vi "ClassPanel.vi"(8 "error in (no error)":errorcluster caption="entrée d'erreur (pas d'erreur)", 11 "BNC845.lvclass":refnum<class "BNC845.lvclass">) -> (0 "error out":errorcluster caption="sortie d'erreur", 3 "BNC845.lvclass Out":refnum<class "BNC845.lvclass">)   [LabVIEW 2019, in "BNC845.lvclass"]
uses:
  BNC845.lvclass
  C:/Programmes Labview/LabscanV1A/DevicesClass/BaseDevice/BaseDevice.lvclass
  BaseDevice/ClassQueueMess.ctl
  BNC845_Func.ctl
  BNC845.lvclass/BNC845.ctl
  BaseDevice/Accessor/GetClassEvent.vi
  <instrlib>/Berkeley Nucleonics 845/Berkeley Nucleonics 845.lvlib
panel:
  in  "Scan Mode":u16(ring) items=["Frequency", "Power"]
  in  "Output En":bool
  in  "Con/Disc.":bool
  in  "FUnits":u16(ring)=1 caption="Units" items=["Hz", "MHz", "GHz"]
  in  "MainProgQ":refnum<queue>
  in  "MainProgQEvent":refnum<user-event>
  in  "Acq":bool
  in  "Stop":bool
  in  "Power":dbl caption="Power(dBm)" format="%#.3f"
  in  "MiseAJour":bool
  in  "Freq(Hz)":dbl=60.0 min=0.01 max=20500000000.0 step=0.01 format="%^#.5e"
  out "Init Program":bool
  # "BNC845"
  # "this MUST labeled with class name"
  # "this MUST be present and labeled \"Stop\" and \"Acq\""
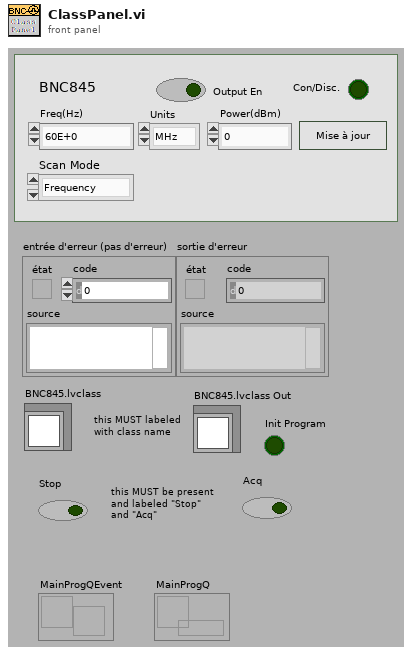
[diagram p1: front panel]
types:
  T1 = typedef "BNC845.lvclass/BNC845_Func.ctl" = enum16{"SetPower (dBm)", "SetFrequency (Hz)"}
  T2 = typedef "ClassQueueMess.ctl" = u16
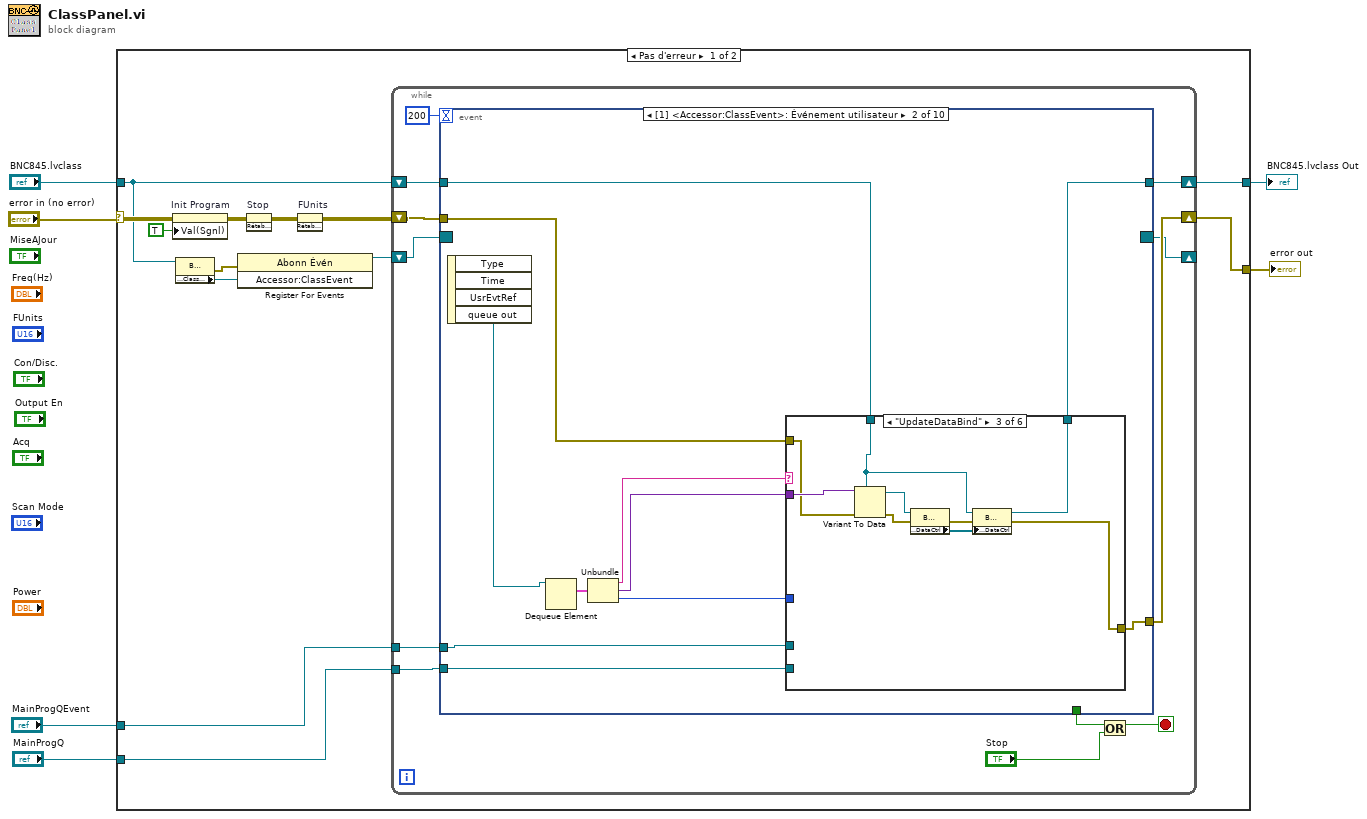
[diagram p0: block diagram]
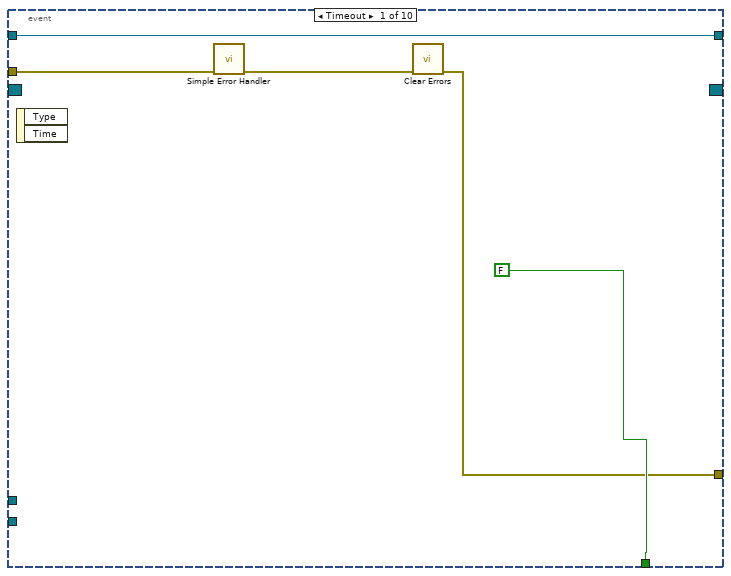
[diagram p2: hidden frame]
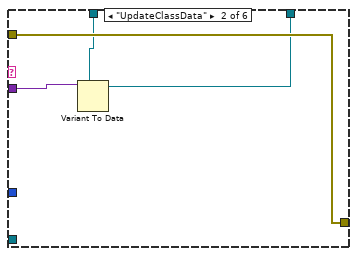
[diagram p4: hidden frame]
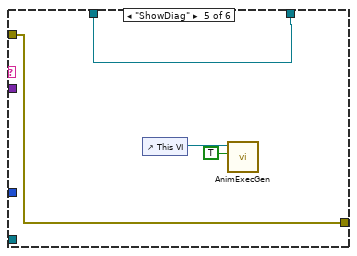
[diagram p6: hidden frame]
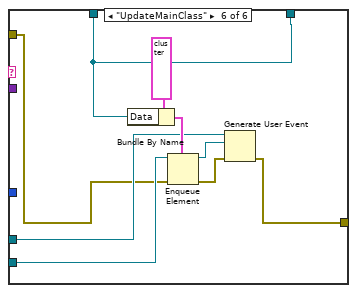
[diagram p7: hidden frame]
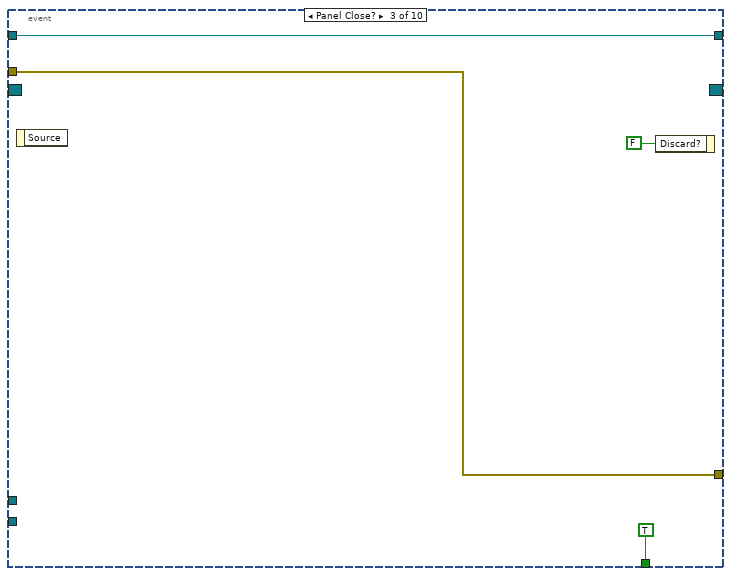
[diagram p8: hidden frame]
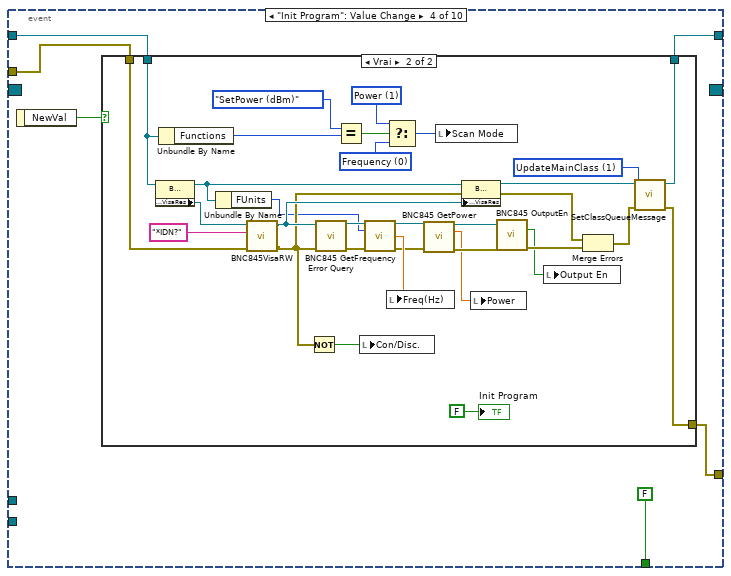
[diagram p9: hidden frame]
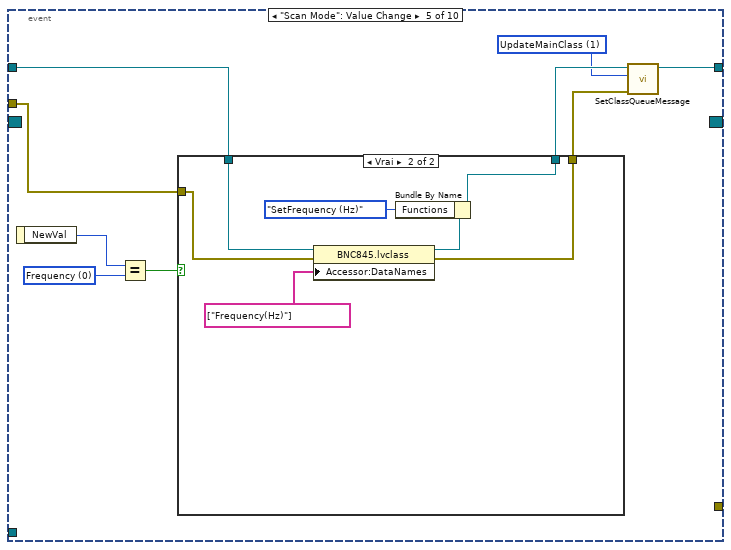
[diagram p11: hidden frame]
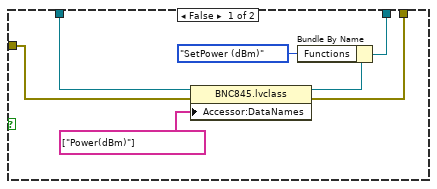
[diagram p12: hidden frame]
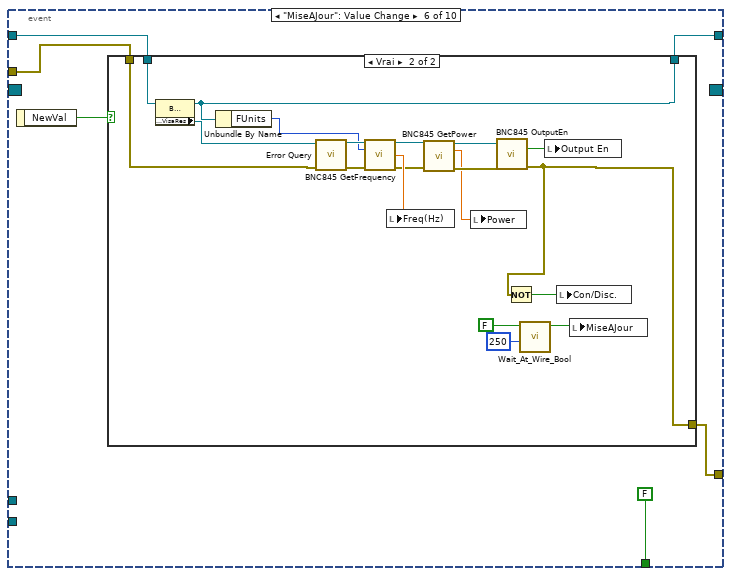
[diagram p13: hidden frame]
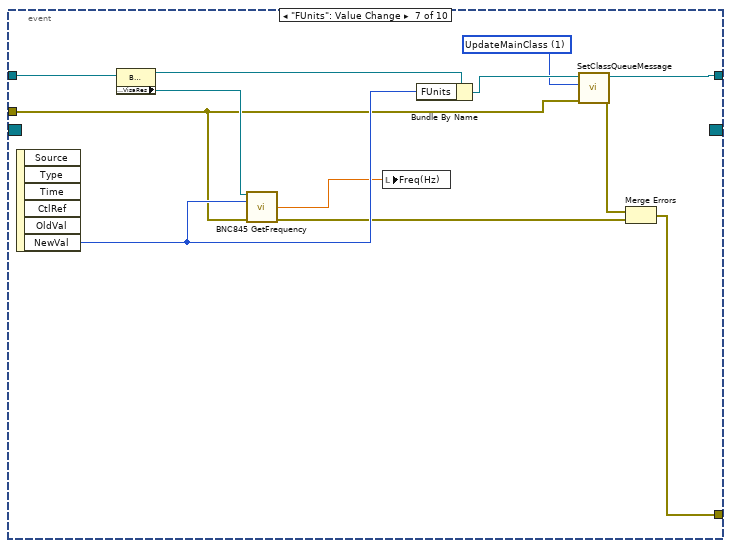
[diagram p15: hidden frame]
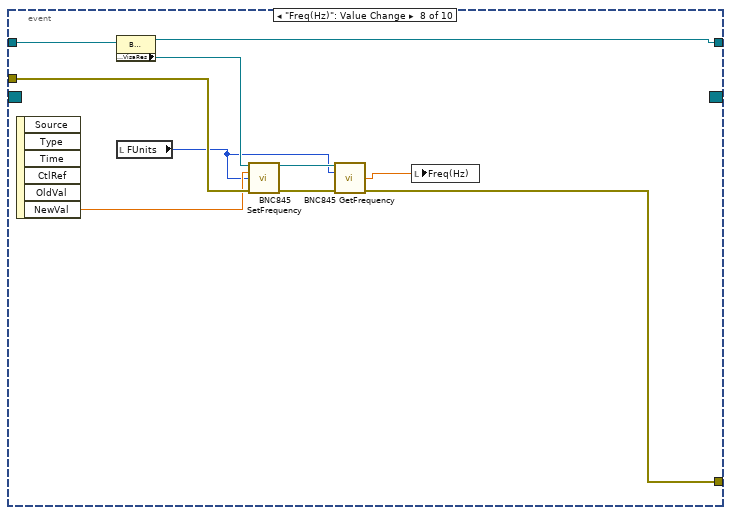
[diagram p16: hidden frame]
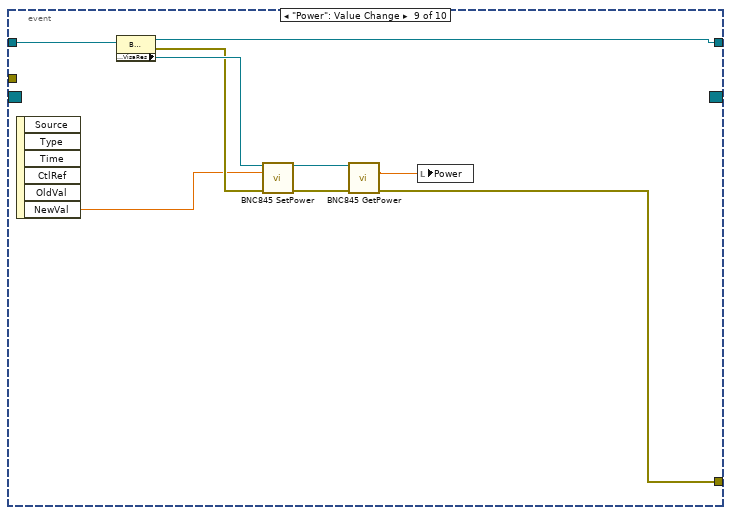
[diagram p17: hidden frame]
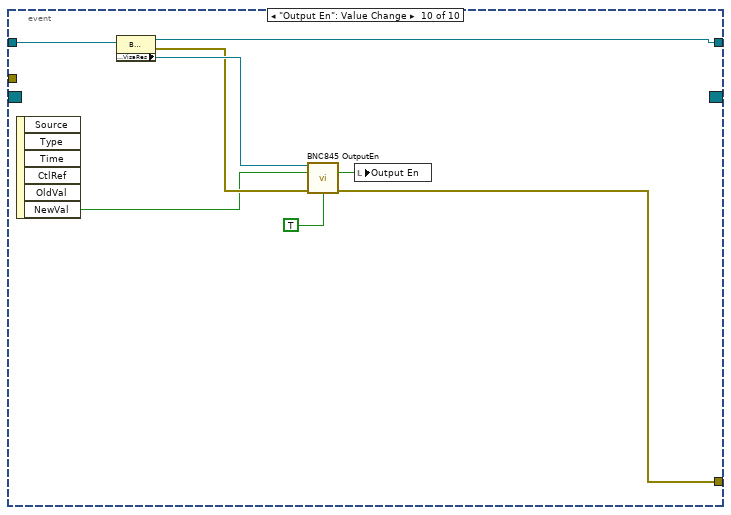
[diagram p18: hidden frame]
diagram:
  n1 = case shown="Pas d'erreur" "error in (no error)" {
    selector: "error in (no error)" -> [w16 w212]
    tunnel: [w19 w212] -> w5
    tunnel: "BNC845.lvclass" -> [w12 w211]
    tunnel: [w17 w211] -> w3
    tunnel: "MainProgQEvent" -> [w10 _]
    tunnel: "MainProgQ" -> [w9 _]
    frame No Error {
      n2 = property on="Init Program" class="Bool (strict)"(error in=w16, "Val(Sgnl)"=TRUE ("Valeur (Signalisation)")) -> (error out=w15:errorcluster)  [unwired: 1 in, 1 out]
      n3 = property class="BNC845.lvclass"(reference=w12) -> (error out=w14:errorcluster, "Accessor:ClassEvent"=w13:refnum<user-event>)  [unwired: 1 in, 1 out]
      n4 = register-events(error in=w14, w13) -> (reference out=w11:refnum<event-registration>)  [unwired: 1 in, 1 out]
      n5 = invoke on="Stop" class="Bool (strict)" method="RétablirValParDéfaut"(error in=w15) -> (error out=w8:errorcluster)  [unwired: 2 in, 2 out]
      n6 = invoke on="FUnits" class="MDér (strict)" method="RétablirValParDéfaut"(error in=w8) -> (error out=w7:errorcluster)  [unwired: 2 in, 2 out]
      n7 = while {
        shift-right: [w29] -> w19
        shift-left: w7 -> [w30]
        shift-right: [w26] -> w17
        shift-left: w12 -> [w28]
        shift-right: [w22] -> _
        shift-left: w11 -> [w23]
        tunnel: w10 -> [w21]
        tunnel: w9 -> [w20]
        stop <- w25 stop-if-true
        n8 = event shown="[1] <Accessor:ClassEvent>: Événement utilisateur" {
          selector: w23 -> [_ _ _ _ _ _ _ _ _ _]
          dyn-events: [_ _ _ _ _ _ _ _ _ _] -> w22
          timeout: 200 -> [_ _ _ _ _ _ _ _ _ _]
          tunnel: w30 -> [w34 w46 w79 w86 w124 w149 w177 w191 _ _]
          tunnel: [w32 w40 w79 w85 _ w148 w175 w185 w199 w208] -> w29
          tunnel: w28 -> [w35 w47 w78 w83 w126 w146 w183 w193 w202 w210]
          tunnel: [FALSE _ TRUE FALSE _ FALSE _ _ _ _] -> w27
          tunnel: [w35 w39 w78 w82 w127 w145 w173 w192 w201 w209] -> w26
          tunnel: w21 -> [_ w38 _ _ _ _ _ _ _ _]
          tunnel: w20 -> [_ w37 _ _ _ _ _ _ _ _]
          event Timeout {
            n9 = event-data() -> ()  [unwired: 1 in, 2 out]
            n10 = call <vilib>:"Simple Error Handler.vi"("error in (no error)"=w34) -> ("error out"=w33:errorcluster)  [unwired: 4 in, 4 out]
            n11 = call <vilib>:"Clear Errors.vi"("error in (no error)"=w33) -> ("error out"=w32:errorcluster)  [unwired: 5 in, 1 out]
          }
          event User Event {
            n12 = event-data() -> ("queue out"=w44:refnum<queue>)  [unwired: 1 in, 3 out]
            n13 = Dequeue Element(queue=w44) -> (element=w45:cluster{"Message":string, "Data":variant, i32})  [unwired: 2 in, 3 out]
            n14 = Unbundle(w45) -> ("Message"=w43:string, "Data"=w42:variant, w41:i32)
            n15 = case shown="\"UpdateDataBind\"" w43 {
              tunnel: w46 -> [w49 w53 w54 w63 w67 w70]
              tunnel: w42 -> [_ w52 w62 _ _ _]
              tunnel: w47 -> [w48 w51 w58 w64 w68 w73]
              tunnel: [w48 w50 w57 w64 w68 w73] -> w39
              tunnel: [w49 w53 w55 w63 w67 w69] -> w40
              tunnel: w41 -> [_ _ _ _ _ _]
              tunnel: w38 -> [_ _ _ _ _ w72]
              tunnel: w37 -> [_ _ _ _ _ w71]
              frame Default {
              }
              frame "UpdateClassData" {
                n16 = Variant To Data(type=w51, Variant=w52) -> (data=w50:refnum<class "BNC845.lvclass">)  [unwired: 1 in, 1 out]
              }
              frame "UpdateDataBind" {
                n17 = Variant To Data(error in=w54, type=w58, Variant=w62) -> (data=w59:refnum<class "BNC845.lvclass">, error out=w56:errorcluster)
                n18 = property class="BNC845.lvclass"(reference=w59, error in=w56) -> (error out=w61:errorcluster, "Accessor:DataCtrl"=w60:refnum<vi>[])  [unwired: 1 out]
                n19 = property class="BNC845.lvclass"(reference=w58, error in=w61, "Accessor:DataCtrl"=w60) -> (reference out=w57:refnum<class "BNC845.lvclass">, error out=w55:errorcluster)
              }
              frame "MeasDone" {
              }
              frame "ShowDiag" {
                n20 = control-ref of="This VI"() -> (w66:refnum<vi>)
                n21 = call <userlib>:"AnimExecGen.vi"("Animer l'exécution ?"=TRUE, "ViRef"=w66) -> ()  [unwired: 9 in, 1 out]
              }
              frame "UpdateMainClass" {
                n22 = Bundle By Name(cluster=cluster{"Message":string, "Data":variant, i32} {"Message"="", "Data"=variant, 0} ("élément"), "Data"=w73) -> (w74:cluster{"Message":string, "Data":variant, i32})
                n23 = Enqueue Element(queue=w71, element=w74, error in (no error)=w70) -> (queue out=w77:refnum<queue>, error out=w76:errorcluster)  [unwired: 1 in, 1 out]
                n24 = Generate User Event(user event=w72, event data cluster=w77, error in=w76) -> (error out=w69:errorcluster)  [unwired: 1 in, 1 out]
              }
            }
          }
          event Panel Close? {
            n25 = event-data() -> ()  [unwired: 1 in, 1 out]
            n26 = event-data("Discard?"=FALSE ("Rejeter ?")) -> ()  [unwired: 1 in, 1 out]
          }
          event "Init Program": Value Change {
            n27 = event-data() -> ("NewVal"=w87:bool)  [unwired: 1 in]
            n28 = case shown="Vrai" w87 {
              tunnel: w86 -> [w89 w119]
              tunnel: [w89 w103] -> w85
              tunnel: w83 -> [w88 w96]
              tunnel: [w88 w108] -> w82
              frame False {
              }
              frame True {
                w90 = u16 0 items=["Frequency", "Power"] ("Scan Mode")
                w91 = u16 1 items=["Frequency", "Power"] ("Scan Mode")
                w107 = T2 1 items=["UpdateClassData", "UpdateMainClass", "UpdateDataBind", "ReInitDevice", "Custom", "ClosePan"] ("Menu déroulant")
                n29 = property class="BNC845.lvclass"(reference=w96) -> (reference out=w111:refnum<class "BNC845.lvclass">, "Accessor:VisaRes"=w120:refnum<visa-resource-name>)  [unwired: 1 in, 1 out]
                n30 = Unbundle By Name(w96) -> ("Functions"=w94:T1)
                n31 = Unbundle By Name(w111) -> ("FUnits"=w110:u16)
                n32 = call <instrlib>:"BNC845VisaRW.vi"("error in (no error)"=w119, "ChaineCom"="*IDN?", "VISA Rsrc"=w120) -> ("error out"=w114:errorcluster, "VISA Rsrc Out"=w115:refnum<visa-resource-name>)  [unwired: 4 in, 2 out]
                n33 = Not(x=w114) -> (.not. x?=w113:bool)
                n34 = call <instrlib>:"Error Query.vi"("VISA resource name"=w115, "error in (no error)"=w114) -> ("VISA resource name out"=w116:refnum<visa-resource-name>, "error out"=w117:errorcluster)  [unwired: 10 in, 2 out]
                n35 = Equal?(x=BNC845_Func."SetPower (dBm)" ("Functions"), y=w94) -> (x = y?=w93:bool)
                n36 = local write "Con/Disc."(w113) -> ()
                n37 = call <instrlib>:"BNC845 GetFrequency.vi"("VISA Rsrc"=w116, "FUnits"=w110, "error in (no error)"=w117) -> ("VISA Rsrc Out"=w101:refnum<visa-resource-name>, "Frequency (Units)"=w112:dbl, "error out"=w102:errorcluster)  [unwired: 9 in, 1 out]
                n38 = Select(t=w91, s=w93, f=w90) -> (s? t:f=w92:u16)
                n39 = local write "Freq(Hz)"(w112) -> ()
                n40 = call <instrlib>:"BNC845 GetPower.vi"("VISA Rsrc"=w101, "error in (no error)"=w102) -> ("VISA Rsrc Out"=w98:refnum<visa-resource-name>, "Power (dBm)"=w99:dbl, "error out"=w100:errorcluster)  [unwired: 11 in]
                n41 = local write "Scan Mode"(w92) -> ()
                n42 = property class="BNC845.lvclass"(reference=w111, error in=w114, "Accessor:VisaRes"=w115) -> (reference out=w106:refnum<class "BNC845.lvclass">, error out=w105:errorcluster)
                n43 = local write "Power"(w99) -> ()
                n44 = call <instrlib>:"BNC845 OutputEn.vi"("VISA Rsrc"=w98, "error in (no error)"=w100) -> ("Enabled"=w97:bool, "error out"=w109:errorcluster)  [unwired: 11 in, 1 out]
                n45 = local write "Output En"(w97) -> ()
                n46 = Merge Errors(w105, w109) -> (w104:errorcluster)
                n47 = call-dynamic "SetClassQueueMessage.vi"("ErrorIn(No Error)"=w104, "Menu déroulant"=w107, "DefaultDev.lvclass"=w106) -> ("sortie d'erreur"=w103:errorcluster, "DefaultDev.lvclass Out"=w108:refnum<class "BNC845.lvclass">)  [unwired: 7 in]
                "Init Program" <- FALSE
              }
            }
          }
          event "Scan Mode": Value Change {
            w122 = T2 1 items=["UpdateClassData", "UpdateMainClass", "UpdateDataBind", "ReInitDevice", "Custom", "ClosePan"] ("Menu déroulant")
            w130 = u16 0 items=["Frequency", "Power"] ("Scan Mode")
            n48 = event-data() -> ("NewVal"=w129:u16)  [unwired: 1 in]
            n49 = Equal?(x=w129, y=w130) -> (x = y?=w128:bool)
            n50 = case shown="Vrai" w128 {
              tunnel: w126 -> [w135 w142]
              tunnel: [w136 w143] -> w125
              tunnel: w124 -> [w132 w141]
              tunnel: [w131 w140] -> w123
              frame False {
                n51 = property class="BNC845.lvclass"(reference=w135, error in=w132, "Accessor:DataNames"=string[] ["Power(dBm)"]) -> (reference out=w134:refnum<class "BNC845.lvclass">, error out=w131:errorcluster)
                n52 = Bundle By Name(cluster=w134, "Functions"=BNC845_Func."SetPower (dBm)") -> (w136:refnum<class "BNC845.lvclass">)
              }
              frame True {
                n53 = property class="BNC845.lvclass"(reference=w142, error in=w141, "Accessor:DataNames"=string[] ["Frequency(Hz)"]) -> (reference out=w139:refnum<class "BNC845.lvclass">, error out=w140:errorcluster)
                n54 = Bundle By Name(cluster=w139, "Functions"=BNC845_Func."SetFrequency (Hz)") -> (w143:refnum<class "BNC845.lvclass">)
              }
            }
            n55 = call-dynamic "SetClassQueueMessage.vi"("ErrorIn(No Error)"=w123, "Menu déroulant"=w122, "DefaultDev.lvclass"=w125) -> ("DefaultDev.lvclass Out"=w127:refnum<class "BNC845.lvclass">)  [unwired: 7 in, 1 out]
          }
          event "MiseAJour": Value Change {
            n56 = event-data() -> ("NewVal"=w150:bool)  [unwired: 1 in]
            n57 = case shown="Vrai" w150 {
              tunnel: w149 -> [w152 w160]
              tunnel: [w152 w158] -> w148
              tunnel: w146 -> [w151 w171]
              tunnel: [w151 w154] -> w145
              frame False {
              }
              frame True {
                n58 = property class="BNC845.lvclass"(reference=w171) -> (reference out=w154:refnum<class "BNC845.lvclass">, "Accessor:VisaRes"=w159:refnum<visa-resource-name>)  [unwired: 1 in, 1 out]
                n59 = Unbundle By Name(w154) -> ("FUnits"=w166:u16)
                n60 = call <instrlib>:"Error Query.vi"("VISA resource name"=w159, "error in (no error)"=w160) -> ("VISA resource name out"=w169:refnum<visa-resource-name>, "error out"=w170:errorcluster)  [unwired: 10 in, 2 out]
                n61 = call <instrlib>:"BNC845 GetFrequency.vi"("VISA Rsrc"=w169, "FUnits"=w166, "error in (no error)"=w170) -> ("VISA Rsrc Out"=w164:refnum<visa-resource-name>, "Frequency (Units)"=w167:dbl, "error out"=w165:errorcluster)  [unwired: 9 in, 1 out]
                n62 = local write "Freq(Hz)"(w167) -> ()
                n63 = call <instrlib>:"BNC845 GetPower.vi"("VISA Rsrc"=w164, "error in (no error)"=w165) -> ("VISA Rsrc Out"=w161:refnum<visa-resource-name>, "Power (dBm)"=w162:dbl, "error out"=w163:errorcluster)  [unwired: 11 in]
                n64 = local write "Power"(w162) -> ()
                n65 = call <instrlib>:"BNC845 OutputEn.vi"("VISA Rsrc"=w161, "error in (no error)"=w163) -> ("Enabled"=w153:bool, "error out"=w158:errorcluster)  [unwired: 11 in, 1 out]
                n66 = Not(x=w158) -> (.not. x?=w168:bool)
                n67 = call <userlib>:"Wait_At_Wire_Bool.vi"("Wait (ms)"=u32 250, "error in (no error)"=FALSE) -> ("error out"=w156:bool)  [unwired: 7 in, 2 out]
                n68 = local write "Output En"(w153) -> ()
                n69 = local write "Con/Disc."(w168) -> ()
                n70 = local write "MiseAJour"(w156) -> ()
              }
            }
          }
          event "FUnits": Value Change {
            w172 = T2 1 items=["UpdateClassData", "UpdateMainClass", "UpdateDataBind", "ReInitDevice", "Custom", "ClosePan"] ("Menu déroulant")
            n71 = event-data() -> ("NewVal"=w180:u16)  [unwired: 1 in, 5 out]
            n72 = property class="BNC845.lvclass"(reference=w183) -> (reference out=w182:refnum<class "BNC845.lvclass">, "Accessor:VisaRes"=w181:refnum<visa-resource-name>)  [unwired: 1 in, 1 out]
            n73 = call <instrlib>:"BNC845 GetFrequency.vi"("VISA Rsrc"=w181, "FUnits"=w180, "error in (no error)"=w177) -> ("Frequency (Units)"=w179:dbl, "error out"=w174:errorcluster)  [unwired: 9 in, 2 out]
            n74 = local write "Freq(Hz)"(w179) -> ()
            n75 = Bundle By Name(cluster=w182, "FUnits"=w180) -> (w178:refnum<class "BNC845.lvclass">)
            n76 = call-dynamic "SetClassQueueMessage.vi"("ErrorIn(No Error)"=w177, "Menu déroulant"=w172, "DefaultDev.lvclass"=w178) -> ("sortie d'erreur"=w176:errorcluster, "DefaultDev.lvclass Out"=w173:refnum<class "BNC845.lvclass">)  [unwired: 7 in]
            n77 = Merge Errors(w176, w174) -> (w175:errorcluster)
          }
          event "Freq(Hz)": Value Change {
            n78 = event-data() -> ("NewVal"=w189:dbl)  [unwired: 1 in, 5 out]
            n79 = property class="BNC845.lvclass"(reference=w193) -> (reference out=w192:refnum<class "BNC845.lvclass">, "Accessor:VisaRes"=w190:refnum<visa-resource-name>)  [unwired: 1 in, 1 out]
            n80 = local read "FUnits"() -> (w187:u16)
            n81 = call <instrlib>:"BNC845 SetFrequency.vi"("VISA Rsrc"=w190, "Frequency (Hz)"=w189, "FUnits"=w187, "error in (no error)"=w191) -> ("VISA Rsrc Out"=w188:refnum<visa-resource-name>, "error out"=w186:errorcluster)  [unwired: 10 in]
            n82 = call <instrlib>:"BNC845 GetFrequency.vi"("VISA Rsrc"=w188, "FUnits"=w187, "error in (no error)"=w186) -> ("Frequency (Units)"=w184:dbl, "error out"=w185:errorcluster)  [unwired: 9 in, 2 out]
            n83 = local write "Freq(Hz)"(w184) -> ()
          }
          event "Power": Value Change {
            n84 = event-data() -> ("NewVal"=w194:dbl)  [unwired: 1 in, 5 out]
            n85 = property class="BNC845.lvclass"(reference=w202) -> (reference out=w201:refnum<class "BNC845.lvclass">, error out=w195:errorcluster, "Accessor:VisaRes"=w197:refnum<visa-resource-name>)  [unwired: 1 in]
            n86 = call <instrlib>:"BNC845 SetPower.vi"("VISA Rsrc"=w197, "Power dBm"=w194, "error in (no error)"=w195) -> ("VISA Rsrc Out"=w196:refnum<visa-resource-name>, "error out"=w198:errorcluster)  [unwired: 11 in]
            n87 = call <instrlib>:"BNC845 GetPower.vi"("VISA Rsrc"=w196, "error in (no error)"=w198) -> ("Power (dBm)"=w200:dbl, "error out"=w199:errorcluster)  [unwired: 11 in, 1 out]
            n88 = local write "Power"(w200) -> ()
          }
          event "Output En": Value Change {
            n89 = event-data() -> ("NewVal"=w205:bool)  [unwired: 1 in, 5 out]
            n90 = property class="BNC845.lvclass"(reference=w210) -> (reference out=w209:refnum<class "BNC845.lvclass">, error out=w206:errorcluster, "Accessor:VisaRes"=w207:refnum<visa-resource-name>)  [unwired: 1 in]
            n91 = call <instrlib>:"BNC845 OutputEn.vi"("VISA Rsrc"=w207, "Output En"=w205, "error in (no error)"=w206, "Set?(F)"=TRUE) -> ("Enabled"=w203:bool, "error out"=w208:errorcluster)  [unwired: 9 in, 1 out]
            n92 = local write "Output En"(w203) -> ()
          }
        }
        n93 = Or(x=w27, y="Stop") -> (x .or. y?=w25:bool)
      }
    }
    frame Error {
    }
  }
  "error out" <- w5
  "BNC845.lvclass Out" <- w3
